vi "TDC_getHbtEventCount.vi"(8 "Error In":errorcluster) -> (0 "Error Out":errorcluster, 1 "Last Rate":dbl=100.0, 2 "Last Count":i32=100, 3 "Total Count":i32=2)   [LabVIEW 2011]
uses:
  tdcbase.dll
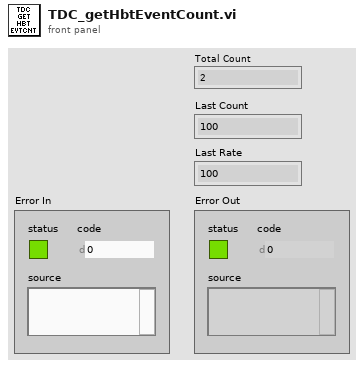
[diagram p1: front panel]
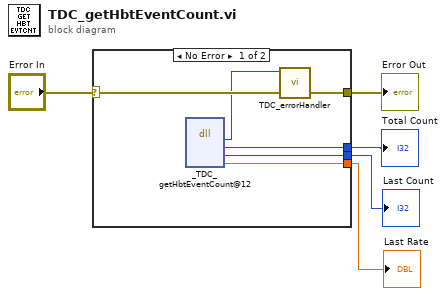
[diagram p0: block diagram]
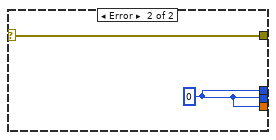
[diagram p2: hidden frame]
diagram:
  n1 = case shown="No Error" "Error In" {
    selector: "Error In" -> [w11 w13]
    tunnel: [w10 w13] -> w4
    tunnel: [w8 w12] -> w3
    tunnel: [w7 w12] -> w2
    tunnel: [w6 w12] -> w1
    frame No Error {
      n2 = dll-call lib="X:/tdcbase.dll" fn="_TDC_getHbtEventCount@12"() -> ("return type"=w9:i32, "totalCnt"=w8:i32, "lastCnt"=w7:i32, "lastRate"=w6:dbl)  [unwired: 6 in, 2 out]
      n3 = call "TDC_errorHandler.vi"("Error In"=w11, "TDC Return Code"=w9) -> ("Error Out"=w10:errorcluster)  [unwired: 9 in]
    }
    frame Error {
      w12 = 0
    }
  }
  "Error Out" <- w4
  "Total Count" <- w3
  "Last Count" <- w2
  "Last Rate" <- w1
